vi "Write configuration.vi"(8 "error in":errorcluster, 10 "configuration":refnum<class "NISE_CEF_serializable configuration.lvclass">, 11 "Modbus Slave editor node in":refnum<class "Modbus Module editor node.lvclass">) -> (0 "error out":errorcluster, 3 "Modbus Slave editor node out":refnum<class "Modbus Module editor node.lvclass">)   [LabVIEW 2013, in "Modbus Module editor node.lvclass"]
doc: "Platypus Framework 1.0.1.65\nNI Systems Engineering - National Instruments"
uses:
  Modbus Module editor node.lvclass
  <vilib>/NI/Configuration Framework/serializable configuration/NISE_CEF_serializable configuration.lvclass
  module/configuration/Modbus Module configuration.lvclass
  Modbus Module editor node.lvclass/Modbus Module editor node.ctl
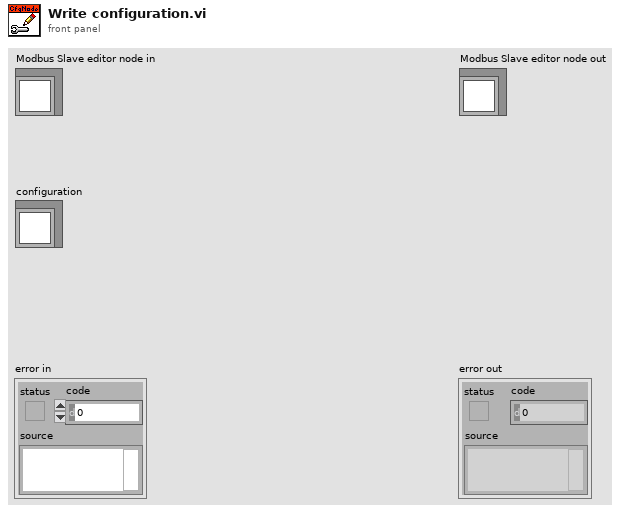
[diagram p1: front panel]
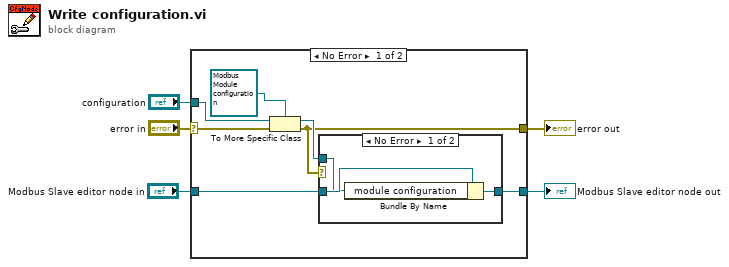
[diagram p0: block diagram]
diagram:
  n1 = case shown="No Error" "error in" {
    selector: "error in" -> [w6 w17]
    tunnel: "Modbus Slave editor node in" -> [w12 w18]
    tunnel: [w11 w18] -> w4
    tunnel: [w7 w17] -> w3
    tunnel: "configuration" -> [w10 _]
    frame No Error {
      n2 = To More Specific Class(target class=refnum<class "Modbus Module configuration.lvclass"> refnum ("module configuration"), reference=w10, error in=w6) -> (specific class reference=w8:refnum<class "Modbus Module configuration.lvclass">, error out=w7:errorcluster)
      n3 = case shown="No Error" w7 {
        tunnel: w12 -> [w15 w16]
        tunnel: [w14 w16] -> w11
        tunnel: w8 -> [w13 _]
        frame No Error {
          n4 = Bundle By Name(cluster=w15, "module configuration"=w13) -> (w14:refnum<class "Modbus Module editor node.lvclass">)
        }
        frame Error {
        }
      }
    }
    frame Error {
    }
  }
  "error out" <- w3
  "Modbus Slave editor node out" <- w4
